vi "Shape Example.vi"() -> ()   [LabVIEW 2020]
uses:
  g_ar_toolkit.image/Image Read Size.ctl
  g_ar_toolkit.feature_detection/Contour Retrieval Modes.ctl
  g_ar_toolkit.feature_detection/Contour Approximation Mode.ctl
  g_ar_toolkit.image/ARGB Colour.ctl
  g_ar_toolkit.image/DrawImageToPictureARGB.vi
  g_ar_toolkit.image/CreateEmptyImageARGB.vi/3321fa97-f432-4e1e-8db9-a0df79aed21b.vi
  g_ar_toolkit.image/ReadImageFileARGB.vi/2358f293-6357-4b7a-bec3-c4e4d03be6e5.vi
  g_ar_toolkit.image/DrawImageToPictureARGB.vi/8cd07b1b-062e-4fe4-9e87-2eb3dc89fe0e.vi
  g_ar_toolkit.image/CreateEmptyImageGreyscale.vi/6598b9e0-8a08-46f5-91fd-ca1b87217137.vi
  g_ar_toolkit.image/ARGBExtractChannel.vi
  g_ar_toolkit.image/ThresholdCore.vi
  g_ar_toolkit.image/DrawImageToPictureGreyscale.vi/9ae995ca-ccda-485c-89ac-02736fde3e8e.vi
  g_ar_toolkit.image/DrawFilledPolyOnImageARGB.vi/e24a04ad-8575-4d64-b8af-da4c51ecb9cd.vi
  g_ar_toolkit.image/ARGBColourToU32.vi
  <vilib>/Utility/error.llb/Error Cluster From Error Code.vi
  g_ar_toolkit.image/CreateEmptyImageARGB.vi
  g_ar_toolkit.image/DrawImageToPictureGreyscale.vi
  g_ar_toolkit.image/ThresholdBinary.vi
  g_ar_toolkit.image/ReadImageFileARGB.vi
  g_ar_toolkit.image/DrawFilledPolyOnImageARGB.vi
  g_ar_toolkit.image/g_ar_toolkit.image.lvlib
  g_ar_toolkit.feature_detection/g_ar_toolkit.feature_detection.lvlib
  g_ar_toolkit.shape/g_ar_toolkit.shape.lvlib
panel:
  out "Input":picture
  out "Thresholded":picture
  out "Draw Contours On Original Image":picture
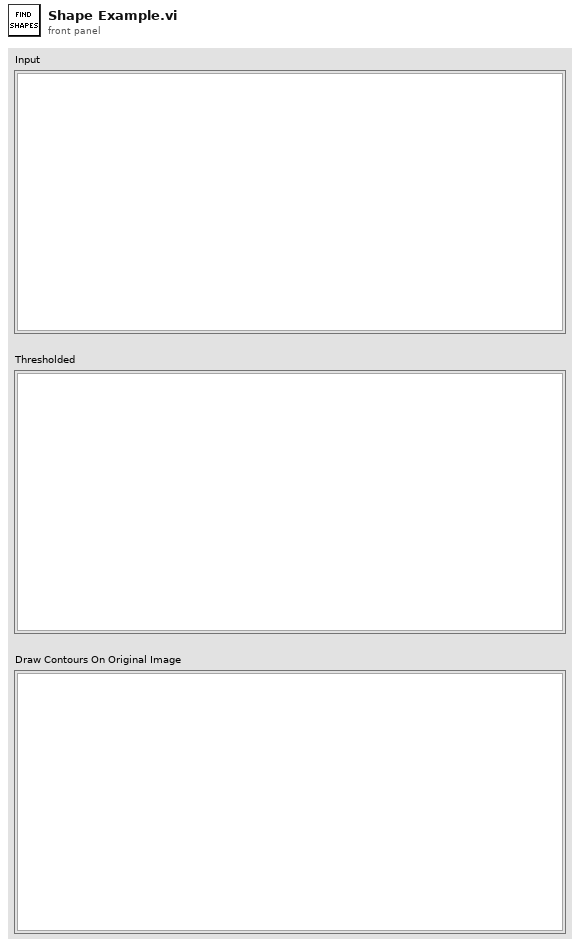
[diagram p1: front panel]
types:
  T1 = typedef "g_ar_toolkit.feature_detection.lvlib/Contour Approximation Mode.ctl" = enum16{"NONE", "SIMPLE", "TC89_L1", "TC89_KCOS"}
  T2 = typedef "g_ar_toolkit.feature_detection.lvlib/Contour Retrieval Modes.ctl" = enum16{"EXTERNAL", "LIST", "CCOMP", "TREE"}
  T3 = typedef "g_ar_toolkit.image.lvlib/Image Read Size.ctl" = enum8{"FULL_SIZE", "REDUCED_2", "REDUCED_4", "REDUCED_8"}
  T4 = typedef "g_ar_toolkit.feature_detection.lvlib/Found Contour.ctl" = cluster{"Points":T5[], "Hierarchy":T6}
  T5 = typedef "g_ar_toolkit.common.lvlib/Image Point (Integer).ctl" = cluster{"x":i32, "y":i32}
  T6 = typedef "g_ar_toolkit.feature_detection.lvlib/Contour Hierarchy.ctl" = cluster{"Previous Contour Index":i32, "Next Contour Index":i32, "First Child Contour Index":i32, "Parent Contour Index":i32}
  T7 = typedef "g_ar_toolkit.image.lvlib/ARGB Colour.ctl" = cluster{"Alpha":u8, "RGB":u32}
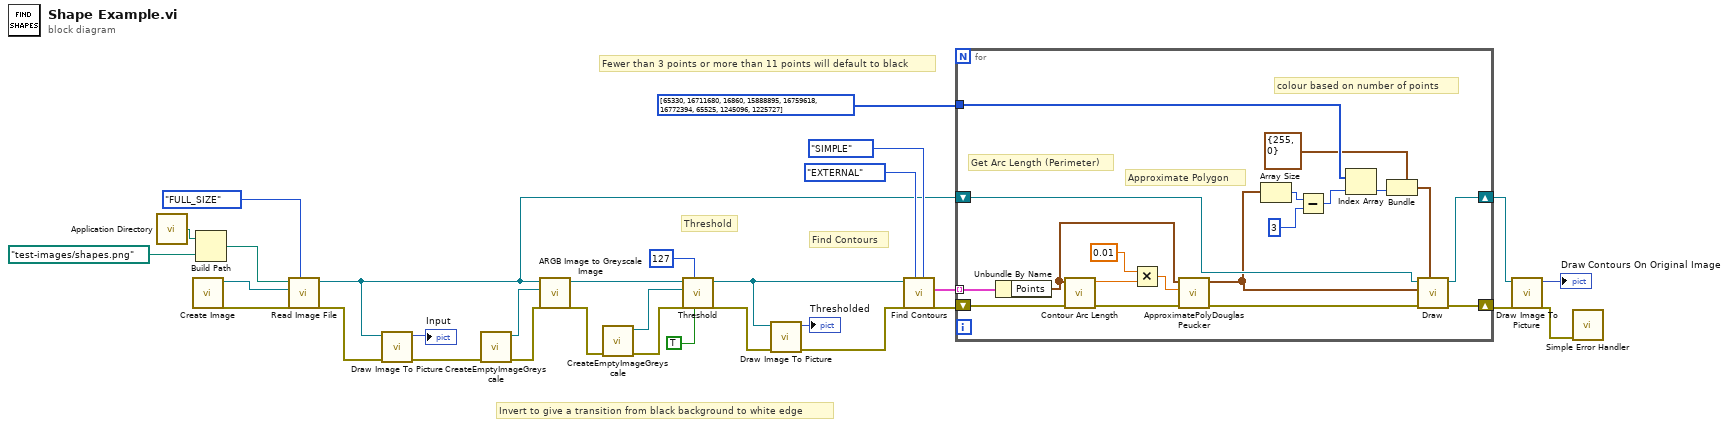
[diagram p0: block diagram]
diagram:
  # "Invert to give a transition from black background to white edge"
  # "Find Contours"
  # "Threshold"
  # "Fewer than 3 points or more than 11 points will default to black"
  n1 = call <vilib>:"Application Directory.vi"() -> ("Application Directory"=w16:path)
  n2 = call-poly "Create Image.vi"() -> ("error out"=w29:errorcluster, "New ARGB Image"=w30:refnum<data-value>)  [unwired: 10 in]
  n3 = Build Path(base path=w16, name or relative path=path "test-images/shapes.png" ("Path")) -> (appended path=w31:path)
  n4 = call-poly "Read Image File.vi"("Image Read Size (Default: FULL_SIZE)"=Image_Read_Size."FULL_SIZE", "error in (no error)"=w29, "ARGB Image Destination"=w30, "Filepath"=w31) -> ("error out"=w7:errorcluster, "ARGB Image Destination (duplicate)"=w8:refnum<data-value>)  [unwired: 6 in]
  n5 = call-poly "Draw Image To Picture.vi"("error in (no error)"=w7, "ARGB Image Source"=w8) -> ("error out"=w6:errorcluster, "Picture"=→"Input":picture)  [unwired: 8 in]
  n6 = call "CreateEmptyImageGreyscale.vi"("error in (no error)"=w6) -> ("error out"=w15:errorcluster, "New Greyscale Image"=w14:refnum<data-value>)  [unwired: 9 in]
  n7 = call "ARGB Image to Greyscale Image.vi"("error in (no error)"=w15, "Greyscale Image Destination"=w14, "ARGB Image Source"=w8) -> ("error out"=w13:errorcluster, "Greyscale Image Destination (Duplicate)"=w12:refnum<data-value>)  [unwired: 7 in]
  n8 = call "CreateEmptyImageGreyscale.vi"("error in (no error)"=w13) -> ("error out"=w26:errorcluster, "New Greyscale Image"=w28:refnum<data-value>)  [unwired: 9 in]
  n9 = call-poly "Threshold.vi"("Invert? (Default: False)"=TRUE, "Threshold"=u8 127, "error in (no error)"=w26, "Threshold Result"=w28, "Greyscale Image-Source"=w12) -> ("error out"=w5:errorcluster, "Threshold Result (duplicate)"=w3:refnum<data-value>)  [unwired: 5 in]
  n10 = call-poly "Draw Image To Picture.vi"("error in (no error)"=w5, "Greyscale Image Source"=w3) -> ("error out"=w4:errorcluster, "Picture"=→"Thresholded":picture)  [unwired: 8 in]
  n11 = call "Find Contours.vi"("Contour Approximation Mode (Default: SIMPLE)"=Contour_Approximation_Mode."SIMPLE", "Contour Retrieval Modes (Default: TREE)"=Contour_Retrieval_Modes."EXTERNAL", "error in (no error)"=w4, "Greyscale Image"=w3) -> ("error out"=w19:errorcluster, "Found Contours"=w18:T4[])  [unwired: 5 in, 1 out]
  n12 = for {
    shift-right: [w49] -> w22
    shift-left: w19 -> [w50]
    tunnel: w18 -> [w45] mode=indexing
    shift-right: [w40] -> w10
    shift-left: w8 -> [w41]
    tunnel: u32[] [65330, 16711680, 16860, 15888895, 16759618, 16772394, 65525, 1245096, 1225727] -> [w37]
    # "Approximate Polygon"
    # "Get Arc Length (Perimeter)"
    # "colour based on number of points"
    n13 = Unbundle By Name(w45) -> ("Points"=w47:T5[])
    n14 = call "Contour Arc Length.vi"("error in (no error)"=w50, "Points in"=w47) -> ("error out"=w44:errorcluster, "Arc Length"=w46:dbl)  [unwired: 8 in]
    n15 = Multiply(x=0.01, y=w46) -> (x*y=w42:dbl)
    n16 = call "ApproximatePolyDouglasPeucker.vi"("error in (no error)"=w44, "Epsilon"=w42, "Points in"=w47) -> ("error out"=w48:errorcluster, "Points out"=w39:T5[])  [unwired: 7 in]
    n17 = Array Size(array=w39) -> (size(s)=w38:i32)
    n18 = Subtract(x=w38, y=3) -> (x-y=w33:i32)
    n19 = Index Array(array=w37, index=w33) -> (element=w34:u32)
    n20 = Bundle(cluster=T7 {"Alpha"=255, "RGB"=0} ("ARGB Colour"), "RGB"=w34) -> (w35:T7)  [unwired: 1 in]
    n21 = call-poly "Draw.vi"("ARGB Colour"=w35, "error in (no error)"=w48, "Points"=w39, "ARGB Image"=w41) -> ("error out"=w49:errorcluster, "ARGB Image (Duplicate)"=w40:refnum<data-value>)  [unwired: 6 in]
  }
  n22 = call-poly "Draw Image To Picture.vi"("error in (no error)"=w22, "ARGB Image Source"=w10) -> ("error out"=w9:errorcluster, "Picture"=→"Draw Contours On Original Image":picture)  [unwired: 8 in]
  n23 = call <vilib>:"Simple Error Handler.vi"("error in (no error)"=w9) -> ()  [unwired: 4 in, 5 out]
